vi "Init.vi"(8 "error in (no error)":errorcluster, 10 "VideoMux Base URL":string) -> (0 "error out":errorcluster, 3 "MuxPanel out":refnum<class "MuxPanel.lvclass">)   [LabVIEW 2022 SP3, in "TouchControl.lvlib" / "MuxPanel.lvclass"]
uses:
  MuxPanel.lvclass
  MuxPanel.lvclass/MuxPanel.ctl
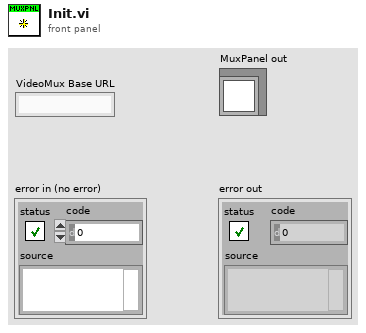
[diagram p1: front panel]
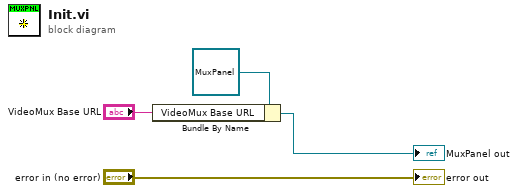
[diagram p0: block diagram]
diagram:
  n1 = Bundle By Name(cluster=refnum<class "MuxPanel.lvclass"> refnum ("MuxPanel in"), "VideoMux Base URL"="VideoMux Base URL") -> (→"MuxPanel out":refnum<class "MuxPanel.lvclass">)
  "error out" <- "error in (no error)"
